vi "ByteArray2HeaderBitArray.vi"(11 "Input Byte Array":u8[](array[numeric])) -> (2 "Header Array":bool[][](array[boolean]), 3 "Found Header":bool)   [LabVIEW 2012]
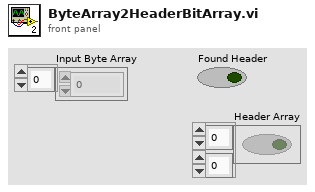
[diagram p1: front panel]
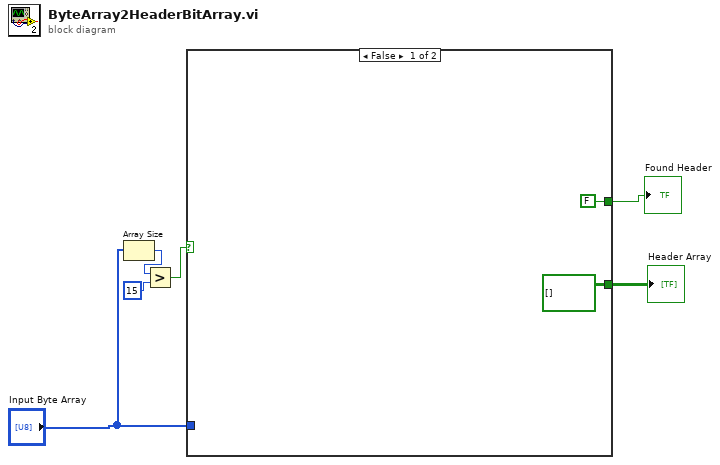
[diagram p0: block diagram]
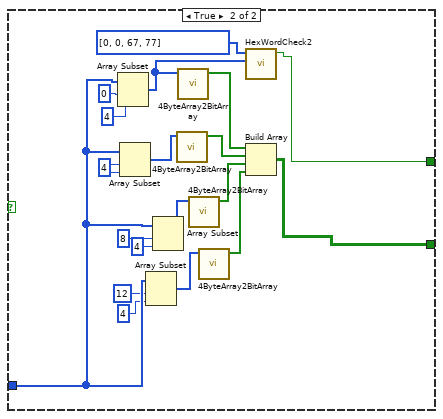
[diagram p2: hidden frame]
diagram:
  n1 = Array Size(array="Input Byte Array") -> (size(s)=w6:i32)
  n2 = Greater?(x=w6, y=15) -> (0:w4:bool)
  n3 = case shown="False" w4 {
    tunnel: "Input Byte Array" -> [_ w27]
    tunnel: [bool[][] [] w10] -> w2
    tunnel: [FALSE ("Boolean") w9] -> w1
    frame False {
    }
    frame True {
      w22 = 4 ("length")
      n4 = Array Subset(array=w27, index=0, length=4) -> (w12:u8[])
      n5 = Array Subset(array=w27, index=w22, length=w22) -> (w26:u8[])
      n6 = Array Subset(array=w27, index=12, length=4) -> (w13:u8[])
      n7 = Array Subset(array=w27, index=8, length=4) -> (w25:u8[])
      n8 = call "4ByteArray2BitArray.vi"("array"=w26) -> ("Array"=w16:bool[])  [unwired: 10 in]
      n9 = call "4ByteArray2BitArray.vi"("array"=w12) -> ("Array"=w17:bool[])  [unwired: 10 in]
      n10 = call "4ByteArray2BitArray.vi"("array"=w25) -> ("Array"=w14:bool[])  [unwired: 10 in]
      n11 = call "4ByteArray2BitArray.vi"("array"=w13) -> ("Array"=w15:bool[])  [unwired: 10 in]
      n12 = call "HexWordCheck2.vi"("array"=w12, "Input Array"=u8[] [0, 0, 67, 77] ("array")) -> ("Boolean"=w9:bool)  [unwired: 9 in]
      n13 = Build Array(w17, w16, w14, w15) -> (w10:bool[][])
    }
  }
  "Found Header" <- w1
  "Header Array" <- w2
